vi "Write Pre-Addressed Messages.vi"(9 "Pre-Addressed Subscribe Msg":refnum<class "Subscribe Msg.lvclass">, 10 "Pre-Addressed Publish Msg":refnum<class "Publish Msg.lvclass">, 11 "IModel in":refnum<class "IModel.lvclass">) -> (3 "IModel out":refnum<class "IModel.lvclass">)   [LabVIEW 2015, in "IModel.lvlib" / "IModel.lvclass"]
doc: "<License>\nCopyright © 2017 Composed Systems, LLC | All rights reserved\nwww.composed.io\n\nAuthor: Ethan Stern <ethan.stern@composed.io>\n\nThis software is provided \"AS IS\" WITHOUT WARRANTIES, either express or implied, AND IS FOR EDUCATIONAL PURPOSES ONLY.\n</License>"
uses:
  IModel.lvclass
  IMediator/IMediator Messages/Publish Msg/Publish Msg.lvclass
  IMediator/IMediator Messages/Subscribe Msg/Subscribe Msg.lvclass
  IModel.lvclass/IModel.ctl
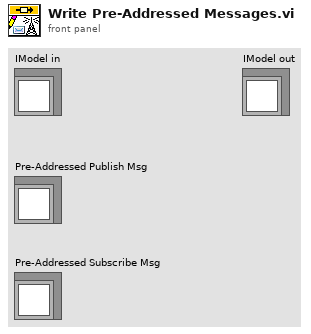
[diagram p1: front panel]
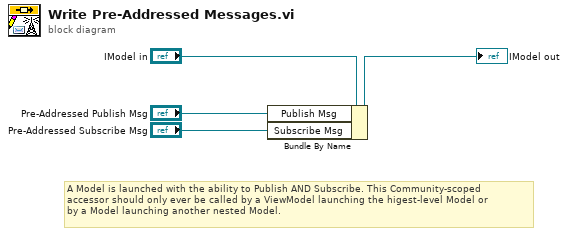
[diagram p0: block diagram]
diagram:
  # "A Model is launched with the ability to Publish AND Subscribe. This Community-scoped\naccessor should only ever be called by a ViewModel launching the higest-level Model or\nby a Model launching another nested Model."
  n1 = Bundle By Name(cluster="IModel in", "Publish Msg"="Pre-Addressed Publish Msg", "Subscribe Msg"="Pre-Addressed Subscribe Msg") -> (→"IModel out":refnum<class "IModel.lvclass">)
